vi "Configure RT StartupVIs.vi"() -> ()   [LabVIEW 2018]
uses:
  <vilib>/Utility/config.llb/Write Key (String).vi
  <vilib>/Utility/config.llb/NI_LVConfig.lvlib
panel:
  out "error out":errorcluster
  # "Run this VI on a LabVIEW Real-Time target to interactively set the \nRTTarget.StartupVIs token in the [lvrt] section of the ni-rt.ini file."
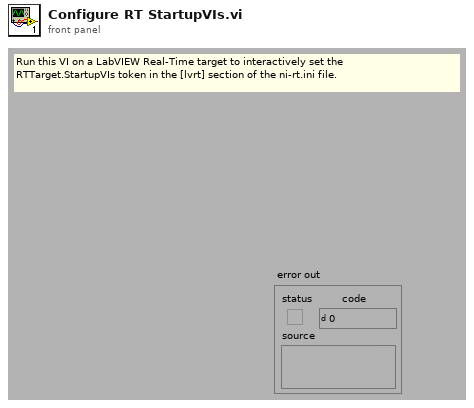
[diagram p1: front panel]
types:
  T1 = typedef "NI_LVConfig.lvlib/Config Data RefNum.ctl" = refnum<k1>
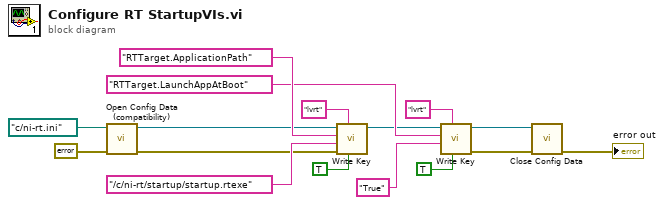
[diagram p0: block diagram]
diagram:
  n1 = call <vilib>:"Open Config Data (compatibility).vi"("error in (no error)"=errorcluster {"status"=FALSE, "code"=0, "source"=""}, "configuration file path"=path "c:/ni-rt.ini") -> ("error out"=w9:errorcluster, "refnum"=w10:T1)  [unwired: 7 in, 1 out]
  n2 = call-poly <vilib>:"Write Key.vi"("write raw string? (F)"=TRUE, "section"="lvrt", "error in (no error)"=w9, "value"="/c/ni-rt/startup/startup.rtexe" ("Current Startup VIs 2"), "key"="RTTarget.ApplicationPath", "refnum"=w10) -> ("refnum out"=w5:T1)  [unwired: 3 in, 2 out]
  n3 = call-poly <vilib>:"Write Key.vi"("write raw string? (F)"=TRUE, "section"="lvrt", "value"="True" ("Current Startup VIs 2"), "key"="RTTarget.LaunchAppAtBoot", "refnum"=w5) -> ("error out"=w2:errorcluster, "refnum out"=w3:T1)  [unwired: 4 in, 1 out]
  n4 = call <vilib>:"Close Config Data.vi"("error in (no error)"=w2, "refnum"=w3) -> ("error out"=→"error out":errorcluster)  [unwired: 8 in, 1 out]
